vi "Edit-dialog.vi"(8 "error in (no error)":errorcluster, 11 "Action in":refnum<class "Move-Relative.lvclass">) -> (0 "error out":errorcluster, 3 "Action out":refnum<class "Move-Relative.lvclass">)   [LabVIEW 2013, in "PowderDeposition.lvlib" / "Move-Relative.lvclass"]
uses:
  Move-Relative.lvclass
  Move-Relative-settings.ctl
  Move-Relative.lvclass/Move-Relative.ctl
panel:
  in  "Cancel":bool
  in  "OK":bool
  in  "Edit dialog":T1
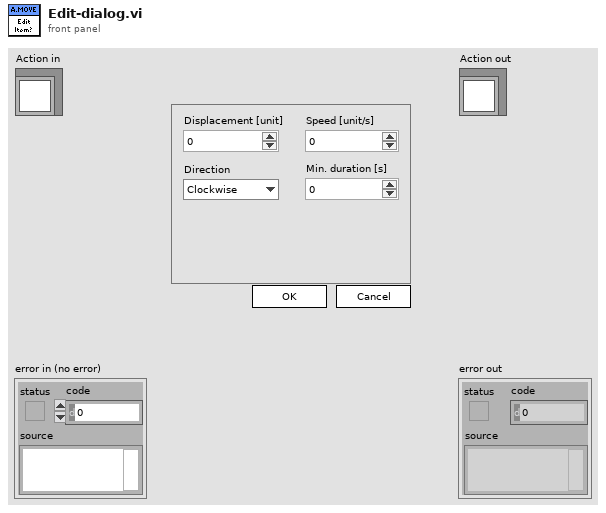
[diagram p1: front panel]
types:
  T1 = typedef "PowderDeposition.lvlib/Move-Relative.lvclass/Move-Relative-settings.ctl" = cluster{"Displacement":dbl, "Speed":dbl, "Direction":enum16{"Clockwise", "Counter-clockwise"}, "Min duration":dbl}
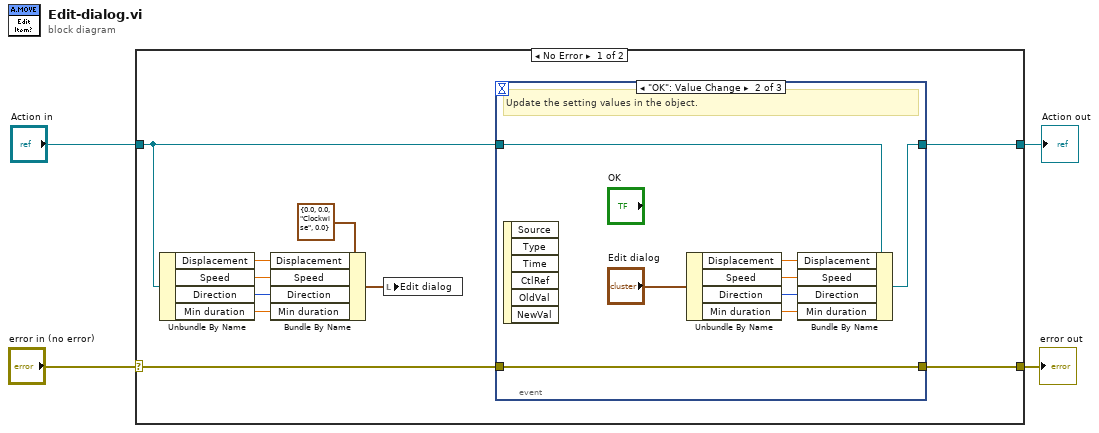
[diagram p0: block diagram]
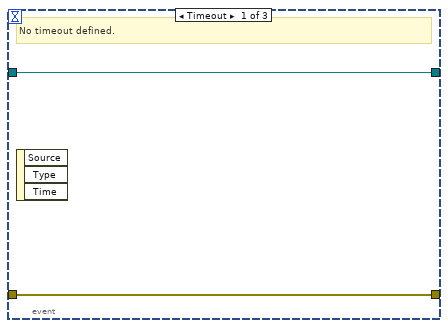
[diagram p2: hidden frame]
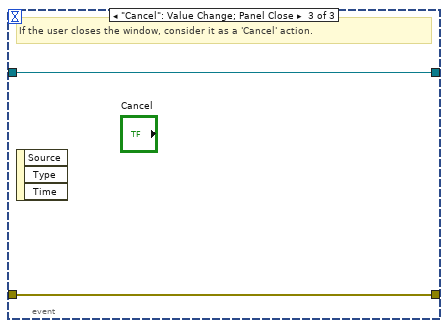
[diagram p3: hidden frame]
diagram:
  n1 = case shown="No Error" "error in (no error)" {
    selector: "error in (no error)" -> [w13 w28]
    tunnel: [w12 w28] -> w3
    tunnel: [w14 w27] -> w1
    tunnel: "Action in" -> [w7 w27]
    frame No Error {
      n2 = Unbundle By Name(w7) -> ("Displacement"=w8:dbl, "Speed"=w9:dbl, "Direction"=w10:enum16{"Clockwise", "Counter-clockwise"}, "Min duration"=w11:dbl)
      n3 = Bundle By Name(cluster=T1 {"Displacement"=0.0, "Speed"=0.0, "Direction"=enum."Clockwise", "Min duration"=0.0} ("Edit dialog"), "Displacement"=w8, "Speed"=w9, "Direction"=w10, "Min duration"=w11) -> (w5:T1)
      n4 = local write "Edit dialog"(w5) -> ()
      n5 = event shown="[1] \"OK\": Value Change" {
        selector: _ -> [_ _ _]
        dyn-events: _ -> [_ _ _]
        timeout: _ -> [_ _ _]
        tunnel: w7 -> [w16 w23 w26]
        tunnel: [w16 w22 w26] -> w14
        tunnel: w13 -> [w15 w24 w25]
        tunnel: [w15 w24 w25] -> w12
        event Timeout {
          # "No timeout defined."
          n6 = event-data() -> ()  [unwired: 1 in, 3 out]
        }
        event "OK": Value Change {
          # "Update the setting values in the object."
          n7 = event-data() -> ()  [unwired: 1 in, 6 out]
          n8 = Unbundle By Name("Edit dialog") -> ("Displacement"=w20:dbl, "Speed"=w19:dbl, "Direction"=w18:enum16{"Clockwise", "Counter-clockwise"}, "Min duration"=w17:dbl)
          n9 = Bundle By Name(cluster=w23, "Displacement"=w20, "Speed"=w19, "Direction"=w18, "Min duration"=w17) -> (w22:refnum<class "Move-Relative.lvclass">)
        }
        event "Cancel": Value Change; Panel Close {
          # "If the user closes the window, consider it as a 'Cancel' action."
          n10 = event-data() -> ()  [unwired: 1 in, 3 out]
        }
      }
    }
    frame Error {
    }
  }
  "error out" <- w3
  "Action out" <- w1
